vi "Dequeue.vi"(7 "PreviewQueue(F)":bool, 8 "error in (no error)":errorcluster, 10 "timeout in ms (-1)":i32=-1, 11 "MessageQueue":refnum<queue>) -> (0 "error out":errorcluster, 1 "Message Data":variant, 2 "Message":string, 3 "MessageQueue":refnum<queue>, 4 "timed out?":bool)   [LabVIEW 2018, in "AcPwrPlugins.lvlib"]
uses:
  AcPwrPlugins/AcPwrPlugins.lvlib
  PublicAPI/Arguments/Messages/clMessage.ctl
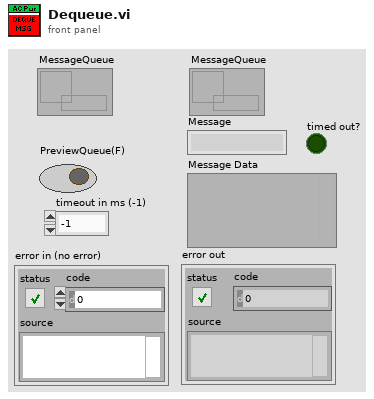
[diagram p1: front panel]
types:
  T1 = typedef "AcPwrPlugins.lvlib/clMessage.ctl" = cluster{"Message":string, "Message Data":variant}
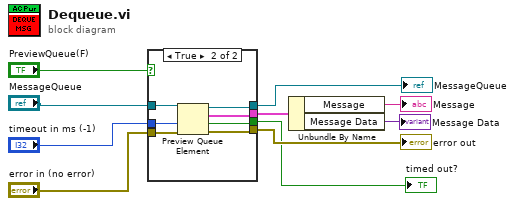
[diagram p0: block diagram]
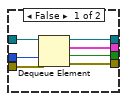
[diagram p2: hidden frame]
diagram:
  n1 = case shown="True" "PreviewQueue(F)" {
    tunnel: [w17 w24] -> w10
    tunnel: "MessageQueue" -> [w16 w22]
    tunnel: "error in (no error)" -> [w15 w23]
    tunnel: [w14 w20] -> w7
    tunnel: [w13 w21] -> w4
    tunnel: "timeout in ms (-1)" -> [w12 w19]
    tunnel: [w11 w18] -> w1
    frame False {
      n2 = Dequeue Element(queue=w16, timeout in ms (-1)=w12, error in (no error)=w15) -> (queue out=w13:refnum<queue>, element=w14:T1, timed out?=w11:bool, error out=w17:errorcluster)
    }
    frame True {
      n3 = Preview Queue Element(queue=w22, timeout in ms (-1)=w19, error in (no error)=w23) -> (queue out=w21:refnum<queue>, element=w20:T1, timed out?=w18:bool, error out=w24:errorcluster)
    }
  }
  "error out" <- w10
  "MessageQueue" <- w4
  "timed out?" <- w1
  n4 = Unbundle By Name(w7) -> ("Message"=→"Message":string, "Message Data"=→"Message Data":variant)
